vi "Process.vi"(8 "error in (no error)":errorcluster, 9 "string refnum":refnum<vi>, 10 "Pound in":refnum<class "Pound.lvclass">, 11 "Qbus in":refnum<class "Qbus.lvclass">) -> (0 "error out":errorcluster)   [LabVIEW 2017, in "TracePointDisplay.lvlib"]
uses:
  <vilib>/addons/InsightCM/Devices/Shared/Common/TracePointDisplay/TracePointDisplay.lvlib
  <vilib>/addons/Qbus/Qbus.lvclass
  <vilib>/NI/Software Watchdog/Pound/Pound.lvclass
  <vilib>/addons/TraceLogger/controls/LogTracepoint.ctl
  <vilib>/addons/TraceLogger/TraceLogger.lvlib
  <vilib>/NI/Software Watchdog/Watchdog/Watchdog.lvclass
  <vilib>/addons/InsightCM/Utilities/GlobalConfiguration/GlobalConfiguration.lvlib
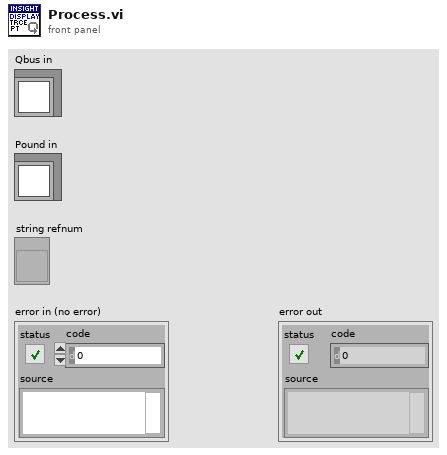
[diagram p1: front panel]
types:
  T1 = typedef "TraceLogger.lvlib/LogTracepoint.ctl" = cluster{"tracepoint":string, "log string":string}
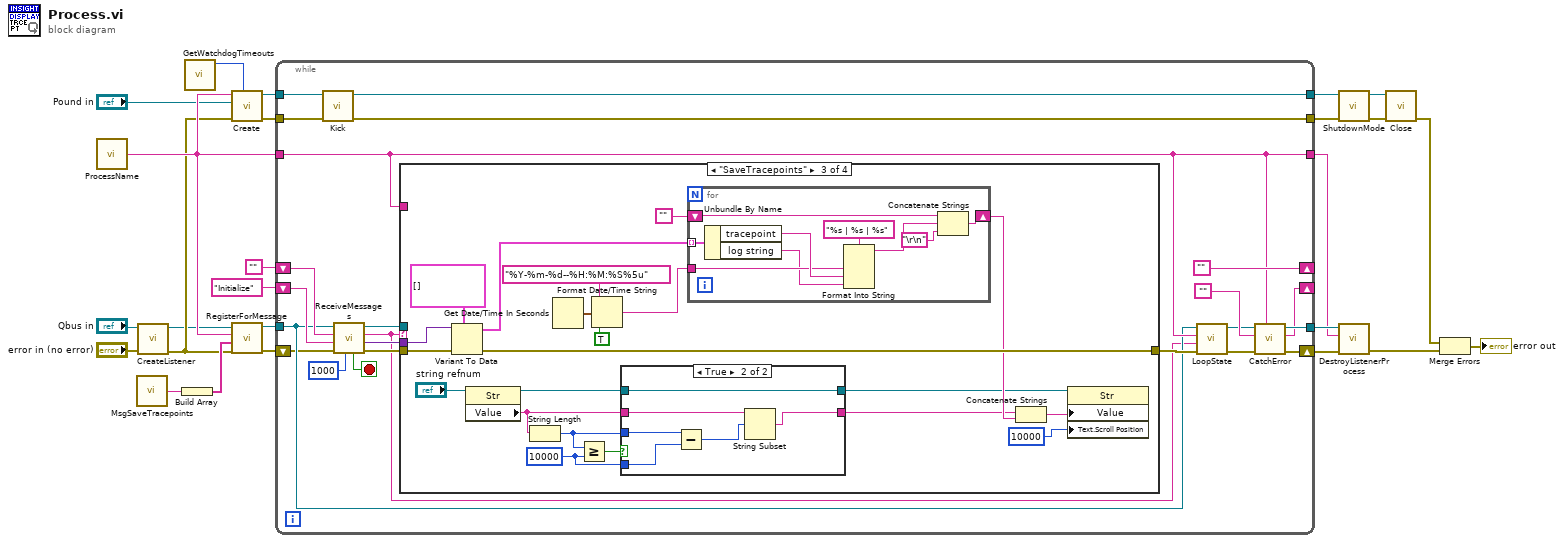
[diagram p0: block diagram]
diagram:
  n1 = call <vilib>:"ProcessName.vi"() -> ("process name"=w17:string)  [unwired: 5 in]
  n2 = call <vilib>:"MsgSaveTracepoints.vi"() -> ("message name"=w6:string)  [unwired: 5 in]
  n3 = call <vilib>:"CreateListener.vi"("error in (no error)"="error in (no error)", "Qbus in"="Qbus in") -> ("error out"=w3:errorcluster, "Qbus out"=w2:refnum<class "Qbus.lvclass">)  [unwired: 8 in]
  n4 = Build Array(w6) -> (w18:string[])
  n5 = call <vilib>:"GetWatchdogTimeouts.vi"() -> ("software timeout"=w1:u32)  [unwired: 10 in, 1 out]
  n6 = call <vilib>:"Create.vi"("Execution Timeout (ms)"=w1, "error in (no error)"=w3, "Pound"="Pound in", "Name"=w17) -> ("error out"=w11:errorcluster, "Watchdog"=w16:refnum<data-value>)  [unwired: 6 in]
  n7 = call <vilib>:"RegisterForMessage.vi"("error in (no error)"=w3, "message names"=w18, "process name"=w17, "Qbus in"=w2) -> ("error in (no error)"=w24:errorcluster, "Qbus out"=w23:refnum<class "Qbus.lvclass">)  [unwired: 6 in]
  n8 = while {
    shift-right: [""] -> _
    shift-left: "" -> [w47]
    tunnel: w23 -> [w36]
    tunnel: w17 -> [w37]
    tunnel: [w41] -> w21
    tunnel: [w37] -> w20
    shift-right: [w39] -> _
    shift-left: "Initialize" -> [w43]
    tunnel: w16 -> [w35]
    tunnel: [w34] -> w13
    tunnel: w11 -> [w33]
    tunnel: [w31] -> w10
    shift-right: [w42] -> w22
    shift-left: w24 -> [w32]
    stop <- w48 stop-if-true
    n9 = call <vilib>:"Kick.vi"("error in (no error)"=w33, "Watchdog"=w35) -> ("error out"=w31:errorcluster, "Watchdog"=w34:refnum<data-value>)  [unwired: 8 in]
    n10 = call <vilib>:"ReceiveMessages.vi"("timeout(1000)"=1000 ("Timeout(100)"), "error in (no error)"=w32, "priority action"=w43, "default action"=w47, "Qbus in"=w36) -> ("error out"=w46:errorcluster, "message value"=w44:variant, "action"=w29:string, "Qbus out"=w30:refnum<class "Qbus.lvclass">, "exit"=w48:bool)  [unwired: 2 in]
    n11 = case shown="\"SaveTracepoints\"" w29 {
      tunnel: w46 -> [w49 w50 w70 w88]
      tunnel: w30 -> [_ _ _ _]
      tunnel: [w49 w50 w70 w88] -> w38
      tunnel: w44 -> [_ _ w69 _]
      tunnel: w37 -> [_ _ _ _]
      frame "", Default {
      }
      frame "Initialize" {
      }
      frame "SaveTracepoints" {
        w52 = 10000 ("y")
        n12 = Variant To Data(error in=w70, type=T1[] [] ("Tracepoints"), Variant=w69) -> (data=w62:T1[])  [unwired: 1 out]
        n13 = property class="Str"(reference="string refnum") -> (reference out=w57:refnum<vi>, "Value"=w56:string)  [unwired: 1 in, 1 out]
        n14 = String Length(string=w56) -> (length=w53:i32)
        n15 = Get Date/Time In Seconds() -> (seconds since 1Jan1904=w65:timestamp)
        n16 = Greater Or Equal?(x=w53, y=w52) -> (x >= y?=w58:bool)
        n17 = Format Date/Time String(time format string (%c)="%Y-%m-%d--%H:%M:%S%5u", seconds (now)=w65, UTC format=TRUE) -> (date/time string=w63:string)
        n18 = case shown="True" w58 {
          tunnel: [w71 w78] -> w54
          tunnel: w57 -> [w71 w78]
          tunnel: [w72 w73] -> w55
          tunnel: w56 -> [w72 w75]
          tunnel: w53 -> [_ w77]
          tunnel: w52 -> [_ w76]
          frame False {
          }
          frame True {
            n19 = Subtract(x=w77, y=w76) -> (x-y=w74:i32)
            n20 = String Subset(string=w75, offset (0)=w74) -> (substring=w73:string)  [unwired: 1 in]
          }
        }
        n21 = for {
          shift-right: [w84] -> w60
          shift-left: "" -> [w86]
          tunnel: w62 -> [w87] mode=indexing
          tunnel: w63 -> [w81]
          n22 = Unbundle By Name(w87) -> ("tracepoint"=w82:string, "log string"=w80:string)
          n23 = Format Into String(format string="%s | %s | %s", w81, w82, w80) -> (resulting string=w79:string)  [unwired: 2 in, 1 out]
          n24 = Concatenate Strings(w86, w79, "\r\n") -> (w84:string)
        }
        n25 = Concatenate Strings(w55, w60) -> (w59:string)
        n26 = property class="Str"(reference=w54, "Value"=w59, "Text.Scroll Position"=u32 10000) -> ()  [unwired: 1 in, 2 out]
      }
      frame "Exit" {
      }
    }
    n27 = call <vilib>:"LoopState.vi"("error in (no error)"=w38, "loop action"=w29, "process name"=w37, "Qbus in"=w36) -> ("error out"=w27:errorcluster, "Qbus out"=w26:refnum<class "Qbus.lvclass">)  [unwired: 6 in]
    n28 = call <vilib>:"CatchError.vi"("source"=w37, "error in (no error)"=w27, "next action in"="", "Qbus in"=w26) -> ("error out"=w42:errorcluster, "next action out"=w39:string, "Qbus out"=w41:refnum<class "Qbus.lvclass">)  [unwired: 5 in]
  }
  n29 = call <vilib>:"ShutdownMode.vi"("error in (no error)"=w10, "Watchdog"=w13) -> ("error out"=w12:errorcluster, "Watchdog"=w14:refnum<data-value>)  [unwired: 8 in]
  n30 = call <vilib>:"DestroyListenerProcess.vi"("error in (no error)"=w22, "process name"=w20, "Qbus in"=w21) -> ("error in (no error)"=w9:errorcluster)  [unwired: 7 in, 1 out]
  n31 = call <vilib>:"Close.vi"("error in (no error)"=w12, "Watchdog"=w14) -> ("error out"=w8:errorcluster)  [unwired: 9 in]
  n32 = Merge Errors(w8, w9) -> (→"error out":errorcluster)
